vi "WriteRegistry - Shell Menu.vi"   [LabVIEW 2017]
uses:
  <vilib>/registry/registry.llb/Registry RtKey.ctl
  <vilib>/registry/registry.llb/Write Registry Value Simple STR.vi
types:
  T1 = enum32{"Invalid", "Standard", "Closed", "Hidden", "Minimized", "Maximized"}
  T2 = typedef "Registry RtKey.ctl" = enum32{"HKEY_CLASSES_ROOT", "HKEY_CURRENT_USER", "HKEY_LOCAL_MACHINE", "HKEY_USERS", "HKEY_PERFORMANCE_DATA", "HKEY_CURRENT_CONFIG", "HKEY_DYN_DATA"}
  T3 = typedef "Registry refnum.ctl" = refnum<k1>
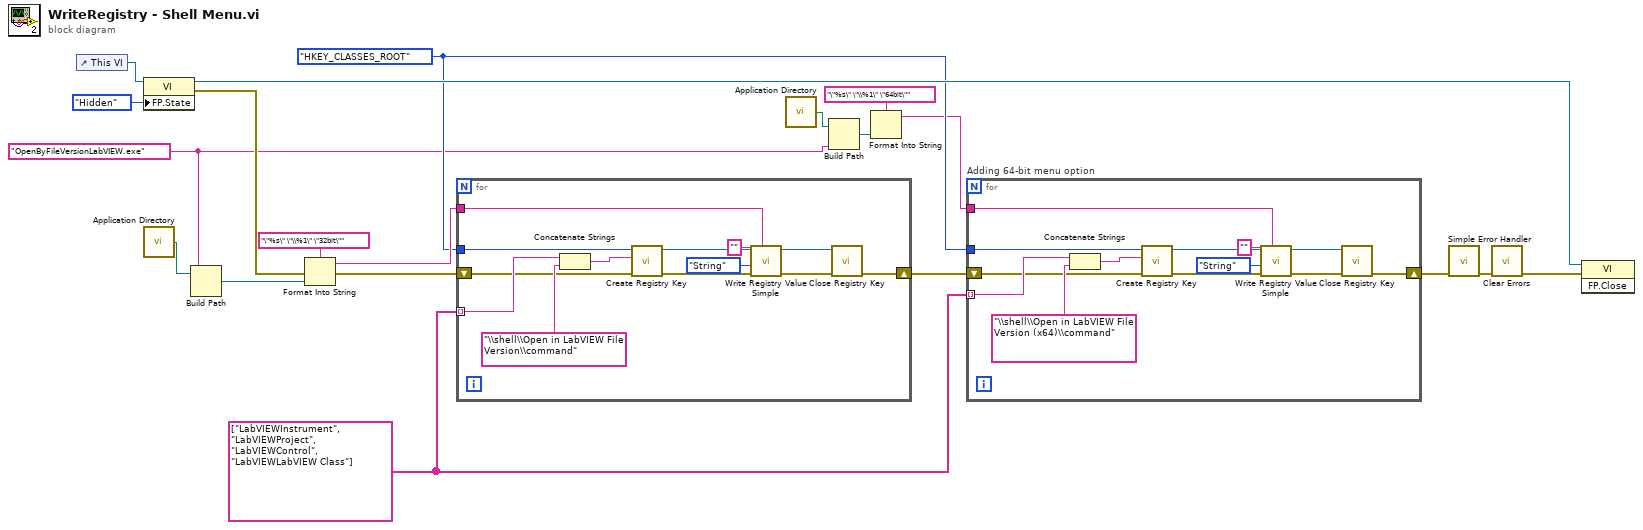
[diagram p0: block diagram]
diagram:
  w1 = "OpenByFileVersionLabVIEW.exe" ("value")
  w11 = string[] ["LabVIEWInstrument", "LabVIEWProject", "LabVIEWControl", "LabVIEWLabVIEW Class"]
  w10 = Registry_RtKey."HKEY_CLASSES_ROOT" ("root key (HKEY_LOCAL_MACHINE)")
  n1 = control-ref of="This VI"() -> (w19:refnum<vi>)
  n2 = property class="VI"(reference=w19, "FP.State"=T1."Hidden" ("Front Panel Window:State")) -> (reference out=w14:refnum<vi>, error out=w5:errorcluster)  [unwired: 1 in]
  n3 = call <vilib>:"Application Directory.vi"() -> ("Application Directory"=w8:path)
  n4 = Build Path(base path=w8, name or relative path=w1) -> (appended path=w20:path)
  n5 = Format Into String(format string="\"%s\" \"\\%1\" \"32bit\"", error in=w5, w20) -> (resulting string=w12:string, error out=w17:errorcluster)  [unwired: 1 in]
  n6 = for {
    tunnel: w12 -> [w22]
    tunnel: w10 -> [w29]
    tunnel: w11 -> [w26] mode=indexing
    shift-right: [w25] -> w13
    shift-left: w17 -> [w24]
    n7 = Concatenate Strings(w26, "\\shell\\Open in LabVIEW File Version\\command" ("string")) -> (w28:string)
    n8 = call <vilib>:"Create Registry Key.vi"("error in (no error)"=w24, "subkey"=w28, "root key (HKEY_LOCAL_MACHINE)"=w29) -> ("error out"=w32:errorcluster, "refnum out"=w33:T3)  [unwired: 6 in, 1 out]
    n9 = call-poly <vilib>:"Write Registry Value Simple.vi"("String/Binary data"=w22, "error in (no error)"=w32, "simple data type"=enum16{"String", "Binary", "DWORD"}."String", "value"="", "refnum"=w33) -> ("error out"=w30:errorcluster, "refnum out"=w31:T3)  [unwired: 3 in]
    n10 = call <vilib>:"Close Registry Key.vi"("error in (no error)"=w30, "refnum"=w31) -> ("error out"=w25:errorcluster)  [unwired: 5 in]
  }
  n11 = call <vilib>:"Application Directory.vi"() -> ("Application Directory"=w3:path)
  n12 = Build Path(base path=w3, name or relative path=w1) -> (appended path=w7:path)
  n13 = Format Into String(format string="\"%s\" \"\\%1\" \"64bit\"", w7) -> (resulting string=w4:string)  [unwired: 2 in, 1 out]
  n14 = for "Adding 64-bit menu option" {
    tunnel: w4 -> [w35]
    tunnel: w10 -> [w42]
    tunnel: w11 -> [w39] mode=indexing
    shift-right: [w38] -> w9
    shift-left: w13 -> [w37]
    n15 = Concatenate Strings(w39, "\\shell\\Open in LabVIEW File Version (x64)\\command" ("string")) -> (w41:string)
    n16 = call <vilib>:"Create Registry Key.vi"("error in (no error)"=w37, "subkey"=w41, "root key (HKEY_LOCAL_MACHINE)"=w42) -> ("error out"=w45:errorcluster, "refnum out"=w46:T3)  [unwired: 6 in, 1 out]
    n17 = call-poly <vilib>:"Write Registry Value Simple.vi"("String/Binary data"=w35, "error in (no error)"=w45, "simple data type"=enum16{"String", "Binary", "DWORD"}."String", "value"="", "refnum"=w46) -> ("error out"=w43:errorcluster, "refnum out"=w44:T3)  [unwired: 3 in]
    n18 = call <vilib>:"Close Registry Key.vi"("error in (no error)"=w43, "refnum"=w44) -> ("error out"=w38:errorcluster)  [unwired: 5 in]
  }
  n19 = call <vilib>:"Simple Error Handler.vi"("error in (no error)"=w9) -> ("error out"=w16:errorcluster)  [unwired: 4 in, 4 out]
  n20 = call <vilib>:"Clear Errors.vi"("error in (no error)"=w16) -> ("error out"=w15:errorcluster)  [unwired: 5 in, 1 out]
  n21 = invoke class="VI" method="FP.Close"(reference=w14, error in=w15) -> ()  [unwired: 1 in, 3 out]
